vi "Create.vi"(8 "error in (no error)":errorcluster caption="错误输入（无错误）", 11 "ProcessClass 输入":refnum<class "ProcessClass.lvclass"> caption="DNL_LabVIEW Object in") -> (0 "error out":errorcluster caption="错误输出", 3 "ProcessClass 输出":refnum<class "ProcessClass.lvclass"> caption="DNL_LabVIEW Object out")   [LabVIEW 2017, in "ProcessClass.lvclass"]
uses:
  ProcessClass.lvclass
  ProcessClass.lvclass/ProcessClass.ctl
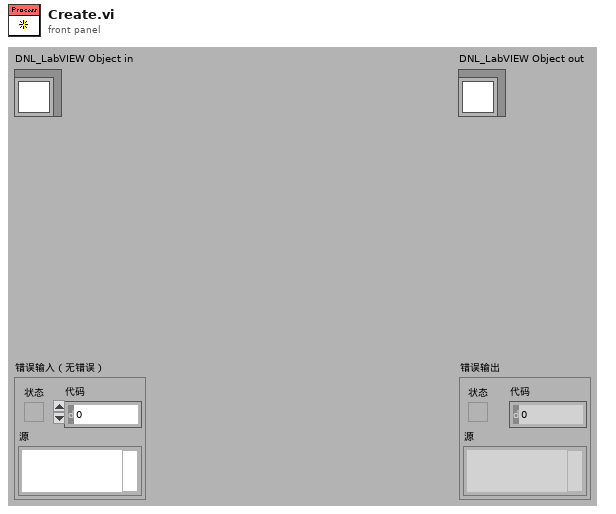
[diagram p1: front panel]
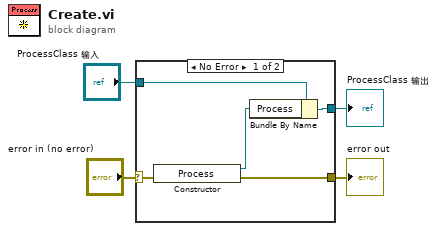
[diagram p0: block diagram]
diagram:
  n1 = case shown="No Error" "error in (no error)" {
    selector: "error in (no error)" -> [w6 w11]
    tunnel: [w5 w11] -> w3
    tunnel: [w7 w10] -> w1
    tunnel: "ProcessClass 输入" -> [w9 w10]
    frame No Error {
      n2 = constructor class="Process"(error in=w6) -> (reference out=w8:refnum<k24>, error out=w5:errorcluster)  [unwired: 2 in, 1 out]
      n3 = Bundle By Name(cluster=w9, "Process"=w8) -> (w7:refnum<class "ProcessClass.lvclass">)
    }
    frame Error {
    }
  }
  "error out" <- w3
  "ProcessClass 输出" <- w1
